vi "QMH Get Next Message from Queue.vi"(7 "error in (no error)":errorcluster, 8 "Termination List ([Exit])":string[](array[string])=["Exit"], 9 "ms timeout (1)":i32=1, 10 "queue in":refnum<queue>) -> (0 "error out":errorcluster, 1 "Next Parameter":string, 2 "Next Message":string, 3 "queue out":refnum<queue>, 4 "Stop QMH":bool)   [LabVIEW 2013, in "QHM.lvlib"]
uses:
  QHM.lvlib
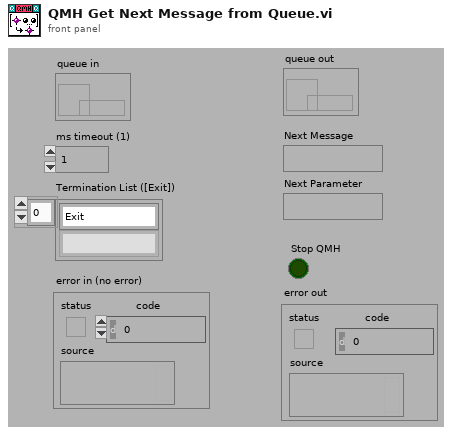
[diagram p1: front panel]
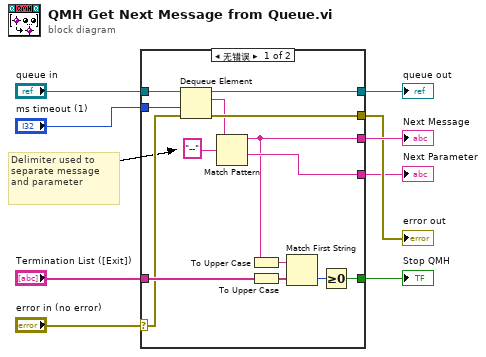
[diagram p0: block diagram]
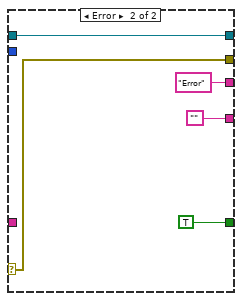
[diagram p2: hidden frame]
diagram:
  # "Delimiter used to\nseparate message\nand parameter"
  n1 = case shown="无错误" "error in (no error)" {
    selector: "error in (no error)" -> [w10 w24]
    tunnel: "queue in" -> [w18 w28]
    tunnel: [w17 w28] -> w3
    tunnel: "Termination List ([Exit])" -> [w23 _]
    tunnel: [w11 "Error"] -> w5
    tunnel: [w21 TRUE] -> w7
    tunnel: "ms timeout (1)" -> [w16 _]
    tunnel: [w15 w24] -> w4
    tunnel: [w12 ""] -> w2
    frame No Error {
      n2 = Dequeue Element(queue=w18, timeout in ms (-1)=w16, error in (no error)=w10) -> (queue out=w17:refnum<queue>, element=w13:string, error out=w15:errorcluster)  [unwired: 1 out]
      n3 = Match Pattern(string=w13, regular expression="--") -> (before substring=w11:string, after substring=w12:string)  [unwired: 1 in, 2 out]
      n4 = To Upper Case(1:w11) -> (0:w20:string)
      n5 = To Upper Case(1:w23) -> (0:w19:string[])
      n6 = Match First String(2:w19, 3:w20) -> (0:w22:i32)  [unwired: 1 out]
      n7 = Greater Or Equal To 0?(x=w22) -> (x >= 0?=w21:bool)
    }
    frame Error {
    }
  }
  "queue out" <- w3
  "Next Message" <- w5
  "Stop QMH" <- w7
  "error out" <- w4
  "Next Parameter" <- w2
